vi "Update Screen - Lunch.vi"(8 "error in (no error)":errorcluster, 11 "Update Screen":T1) -> (0 "error out":errorcluster)   [LabVIEW 2016]
uses:
  Update Screen.ctl
  <vilib>/addons/Display/_Lib/Typedefs/cRIO_Display_Typedefs_DisplayMode.ctl
  <vilib>/addons/Display/_Lib/Typedefs/cRIO_Display_Typedefs_StringConfig.ctl
  <vilib>/addons/Display/_Lib/Typedefs/cRIO_Display_Typedefs_Fonts.ctl
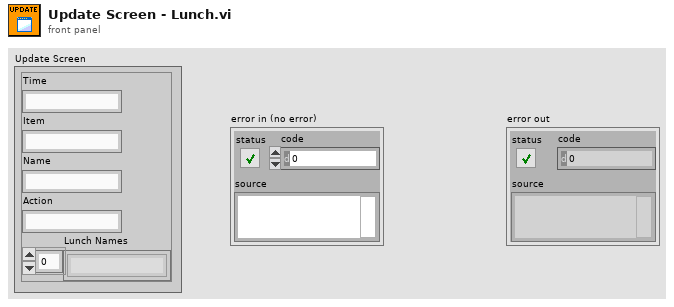
[diagram p1: front panel]
types:
  T1 = typedef "Update Screen.ctl" = cluster{"Time":string, "Item":string, "Name":string, "Action":string, "Lunch Names":string[]}
  T2 = typedef "cRIO_Display_Typedefs_StringConfig.ctl" = cluster{"Column":u8, "Row":u8, "StringColor":u32, "Fontsize":T3}
  T3 = typedef "cRIO_Display_Typedefs_Fonts.ctl" = enum8{"Small", "Medium", "Large", "XLarge"}
  T4 = typedef "cRIO_Display_Typedefs_DisplayMode.ctl" = enum16{"Landscape", "Landscape Rotated", "Portrait", "Portrait Rotated"}
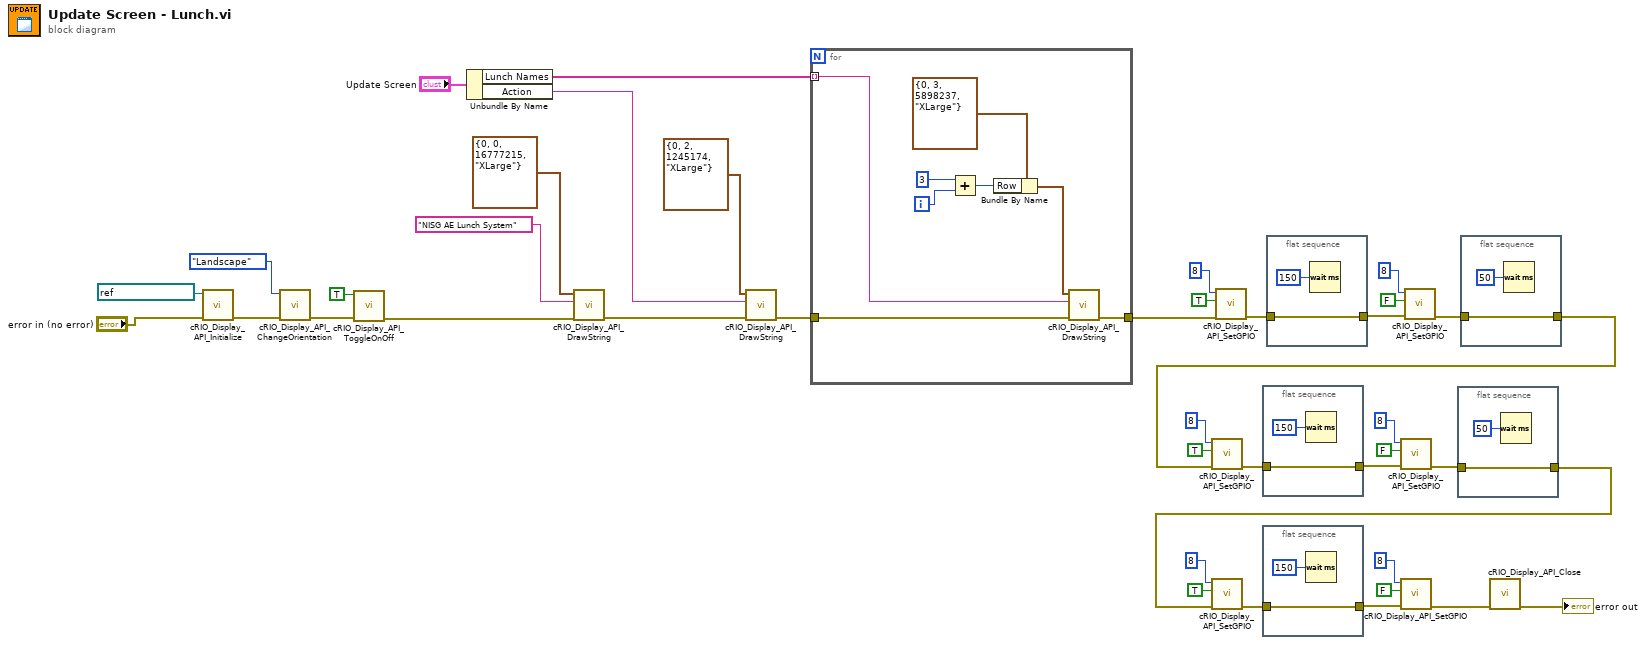
[diagram p0: block diagram]
diagram:
  n1 = call <vilib>:"cRIO_Display_API_Initialize.vi"("error in"="error in (no error)", "cRIODisplay Port"=refnum<visa-resource-name> "ASRL1::INSTR") -> ("error out"=w39:errorcluster)  [unwired: 9 in]
  n2 = call <vilib>:"cRIO_Display_API_ChangeOrientation.vi"("error in"=w39, "DisplayMode"=cRIO_Display_Typedefs_DisplayMode."Landscape") -> ("error out"=w30:errorcluster)  [unwired: 9 in]
  n3 = call <vilib>:"cRIO_Display_API_ToggleOnOff.vi"("error in"=w30, "On/Off"=TRUE) -> ("error out"=w28:errorcluster)  [unwired: 9 in]
  n4 = Unbundle By Name("Update Screen") -> ("Lunch Names"=w19:string[], "Action"=w20:string)
  n5 = call <vilib>:"cRIO_Display_API_DrawString.vi"("error in"=w28, "String"="NISG AE Lunch System", "StringConfig"=T2 {"Column"=0, "Row"=0, "StringColor"=16777215, "Fontsize"=enum."XLarge"}) -> ("error out"=w35:errorcluster)  [unwired: 8 in]
  n6 = call <vilib>:"cRIO_Display_API_DrawString.vi"("error in"=w35, "String"=w20, "StringConfig"=T2 {"Column"=0, "Row"=2, "StringColor"=1245174, "Fontsize"=enum."XLarge"}) -> ("error out"=w37:errorcluster)  [unwired: 8 in]
  n7 = for {
    tunnel: w37 -> [w48]
    tunnel: w19 -> [w42] mode=indexing
    tunnel: [w41] -> w18
    i -> [w45]
    n8 = Add(x=u8 3 ("Row"), y=w45) -> (x+y=w44:i32)
    n9 = Bundle By Name(cluster=T2 {"Column"=0, "Row"=3, "StringColor"=5898237, "Fontsize"=enum."XLarge"} ("StringConfig"), "Row"=w44) -> (w43:T2)
    n10 = call <vilib>:"cRIO_Display_API_DrawString.vi"("error in"=w48, "String"=w42, "StringConfig"=w43) -> ("error out"=w41:errorcluster)  [unwired: 8 in]
  }
  n11 = call <vilib>:"cRIO_Display_API_SetGPIO.vi"("error in"=w2, "GPIO State"=TRUE, "GPIO Pin"=u8 8) -> ("error out"=w16:errorcluster)  [unwired: 8 in]
  n12 = call <vilib>:"cRIO_Display_API_SetGPIO.vi"("error in"=w1, "GPIO State"=TRUE, "GPIO Pin"=u8 8) -> ("error out"=w7:errorcluster)  [unwired: 8 in]
  n13 = call <vilib>:"cRIO_Display_API_SetGPIO.vi"("error in"=w18, "GPIO State"=TRUE, "GPIO Pin"=u8 8) -> ("error out"=w23:errorcluster)  [unwired: 8 in]
  n14 = flat-sequence {
    tunnel: w16 -> [w49]
    tunnel: [w49] -> w17
    frame #0 {
      n15 = Wait (ms)(milliseconds to wait=u32 150) -> ()  [unwired: 1 out]
    }
  }
  n16 = flat-sequence {
    tunnel: w7 -> [w51]
    tunnel: [w51] -> w6
    frame #0 {
      n17 = Wait (ms)(milliseconds to wait=u32 150) -> ()  [unwired: 1 out]
    }
  }
  n18 = flat-sequence {
    tunnel: w23 -> [w53]
    tunnel: [w53] -> w22
    frame #0 {
      n19 = Wait (ms)(milliseconds to wait=u32 150) -> ()  [unwired: 1 out]
    }
  }
  n20 = call <vilib>:"cRIO_Display_API_SetGPIO.vi"("error in"=w17, "GPIO State"=FALSE, "GPIO Pin"=u8 8) -> ("error out"=w3:errorcluster)  [unwired: 8 in]
  n21 = call <vilib>:"cRIO_Display_API_SetGPIO.vi"("error in"=w6, "GPIO State"=FALSE, "GPIO Pin"=u8 8) -> ("error out"=w5:errorcluster)  [unwired: 8 in]
  n22 = call <vilib>:"cRIO_Display_API_SetGPIO.vi"("error in"=w22, "GPIO State"=FALSE, "GPIO Pin"=u8 8) -> ("error out"=w4:errorcluster)  [unwired: 8 in]
  n23 = flat-sequence {
    tunnel: w3 -> [w55]
    tunnel: [w55] -> w1
    frame #0 {
      n24 = Wait (ms)(milliseconds to wait=u32 50) -> ()  [unwired: 1 out]
    }
  }
  n25 = flat-sequence {
    tunnel: w4 -> [w57]
    tunnel: [w57] -> w2
    frame #0 {
      n26 = Wait (ms)(milliseconds to wait=u32 50) -> ()  [unwired: 1 out]
    }
  }
  n27 = call <vilib>:"cRIO_Display_API_Close.vi"("error in"=w5) -> ("error out"=→"error out":errorcluster)  [unwired: 10 in]
